vi "Configure Serial Port.vi"(6 "Parity (0: None)":i32(ring) items=["None", "Even", "Odd"], 7 "Flow Control (0: None)":i32(ring) items=["None", "Hardware"], 8 "error in (no error)":errorcluster, 9 "Data Bits (1: 8)":i32(ring)=1 items=["7", "8"], 10 "Baud Rate (5: 9600)":i32(ring)=5 items=["300", "600", "1200", "2400", "4800", "9600", "19200", "38400", "57600", "115200"], 11 "VISA resource name":refnum<visa-resource-name>) -> (0 "error out":errorcluster, 3 "VISA resource name out":refnum<visa-resource-name>)   [LabVIEW 2019, in "Keithley 2600 Series.lvlib"]
doc: "Configures the basic settings for serial port.\n\n<b>Note:</b>\nThis VI is not available on the model 2606B."
uses:
  Keithley 2600 Series.lvlib
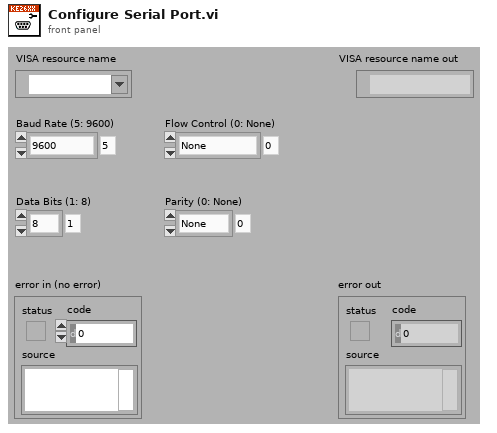
[diagram p1: front panel]
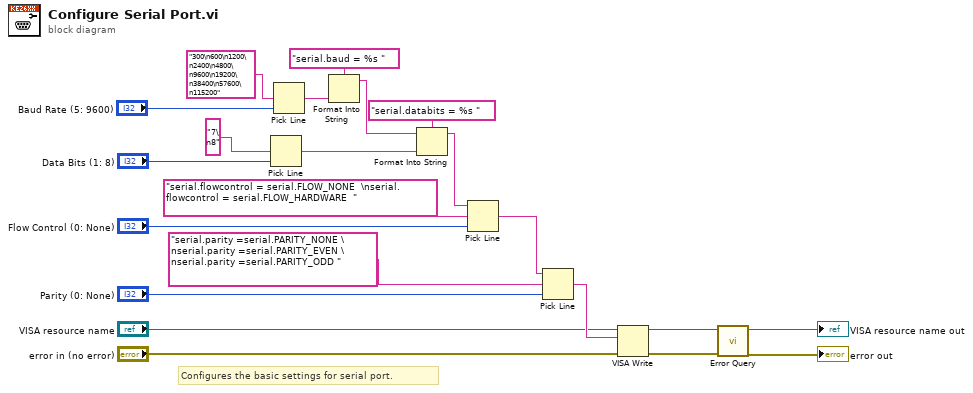
[diagram p0: block diagram]
diagram:
  # "Configures the basic settings for serial port."
  n1 = Pick Line(multi-line string="7\n8", line index="Data Bits (1: 8)") -> (output string=w1:string)  [unwired: 1 in]
  n2 = Pick Line(multi-line string="300\n600\n1200\n2400\n4800\n9600\n19200\n38400\n57600\n115200", line index="Baud Rate (5: 9600)") -> (output string=w5:string)  [unwired: 1 in]
  n3 = Format Into String(format string="serial.baud = %s ", w5) -> (resulting string=w21:string)  [unwired: 2 in, 1 out]
  n4 = Format Into String(format string="serial.databits = %s ", initial string=w21, w1) -> (resulting string=w17:string)  [unwired: 1 in, 1 out]
  n5 = Pick Line(string ("")=w17, multi-line string="serial.flowcontrol = serial.FLOW_NONE  \nserial.flowcontrol = serial.FLOW_HARDWARE  ", line index="Flow Control (0: None)") -> (output string=w14:string)
  n6 = Pick Line(string ("")=w14, multi-line string="serial.parity =serial.PARITY_NONE \nserial.parity =serial.PARITY_EVEN \nserial.parity =serial.PARITY_ODD ", line index="Parity (0: None)") -> (output string=w13:string)
  n7 = VISA Write(VISA resource name="VISA resource name", write buffer=w13, error in (no error)="error in (no error)") -> (VISA resource name out=w10:refnum<visa-resource-name>, error out=w9:errorcluster)  [unwired: 1 out]
  n8 = call "Error Query.vi"("error in (no error)"=w9, "VISA resource name"=w10) -> ("error out"=→"error out":errorcluster, "VISA resource name out"=→"VISA resource name out":refnum<visa-resource-name>)  [unwired: 6 in, 2 out]
